vi "callback_Done.vi"() -> ()   [LabVIEW 2016]
panel:
  out "Z Motor Reference":refnum<k7>
  out "Y Motor Reference":refnum<k7>
  out "X Motor Reference":refnum<k7>
  out "Z Motor done":bool
  out "Y Motor done":bool
  out "X Motor done":bool
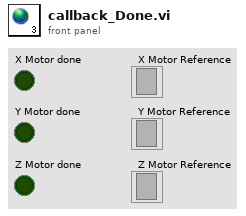
[diagram p1: front panel]
diagram:
